vi "XboxInput.vi"(7 "error in (no error)":errorcluster, 9 "Y In":i16(slide)=50 scale=0.0..100.0, 10 "X In":i16(slide)=50 scale=0.0..100.0) -> (0 "error out":errorcluster, 2 "Y Out":i16(slide) scale=0.0..100.0, 3 "X Out":i16(slide) scale=0.0..100.0)   [LabVIEW 2016]
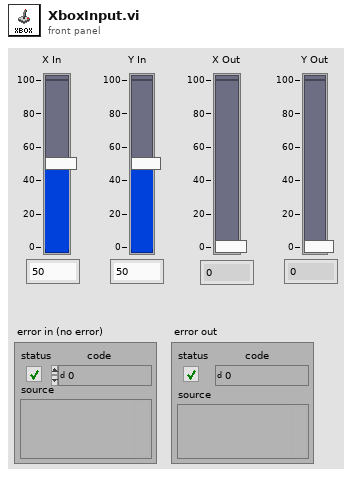
[diagram p1: front panel]
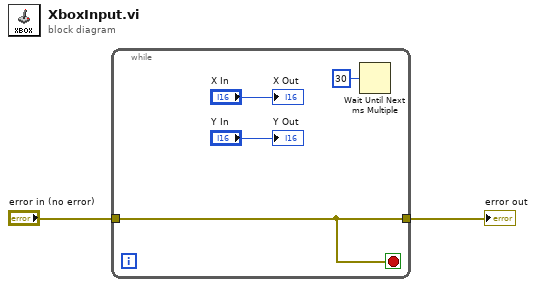
[diagram p0: block diagram]
diagram:
  n1 = while {
    tunnel: [w3] -> w2
    tunnel: "error in (no error)" -> [w3]
    stop <- w3 stop-if-true
    n2 = Wait Until Next ms Multiple(millisecond multiple=u32 30) -> ()  [unwired: 1 out]
    "X Out" <- "X In"
    "Y Out" <- "Y In"
  }
  "error out" <- w2
